vi "Create Event Topics_Latest.vi"() -> (0 "error out":errorcluster, 3 "appended array":string[][](array[string]))   [LabVIEW 2014]
uses:
  <vilib>/National Instruments/NI Amazon Web Services (AWS) Toolkit for LabVIEW/S3/vi source/Typedefs/AMZ_S3_AWS Credentials.ctl
  <vilib>/National Instruments/NI Amazon Web Services (AWS) Toolkit for LabVIEW/SNS/VI Source/Public Typedefs/AWS_SNS CreateTopicParameters.ctl
  <vilib>/National Instruments/NI Amazon Web Services (AWS) Toolkit for LabVIEW/SNS/VI Source/Public Typedefs/AWS_SNS SetTopicAttributes.ctl
  <vilib>/Utility/file.llb/Read From Spreadsheet File (string).vi
  <vilib>/National Instruments/NI Amazon Web Services (AWS) Toolkit for LabVIEW/SNS/VI Source/AWS SNS Class/AWS_SNS.lvclass
  <vilib>/National Instruments/NI Amazon Web Services (AWS) Toolkit for LabVIEW/S3/vi source/LV Interface for Amazon S3.lvlib
  <vilib>/National Instruments/NI Amazon Web Services (AWS) Toolkit for LabVIEW/SNS/VI Source/AWS_SNS.lvlib
panel:
  out "TopicArn":string
  out "resulting string":string
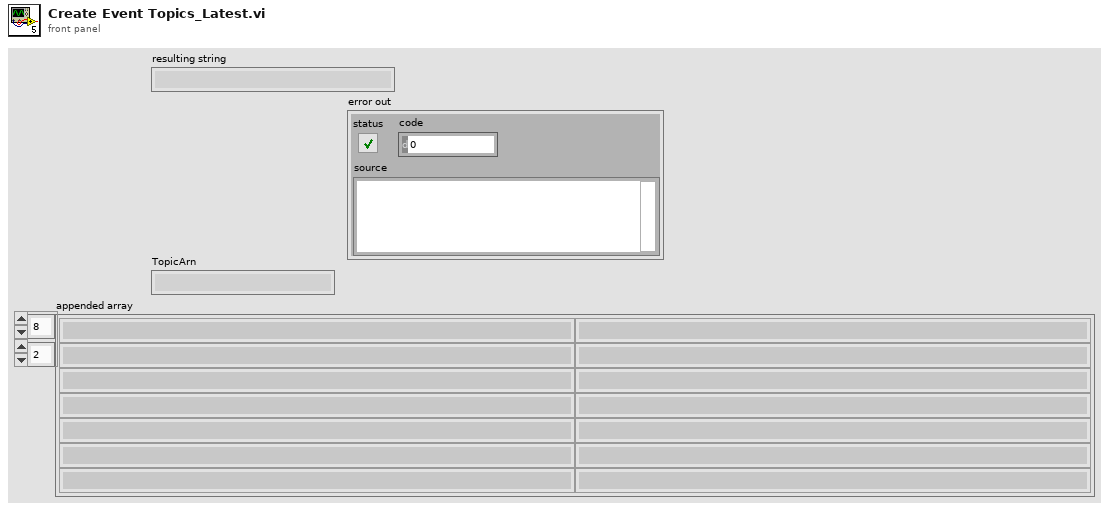
[diagram p1: front panel]
types:
  T1 = typedef "AWS_SNS.lvlib/AWS_SNS CreateTopicParameters.ctl" = string
  T2 = typedef "LV Interface for Amazon S3.lvlib/AMZ_S3_AWS Credentials.ctl" = cluster{"Access Key":string, "Secret Key":string}
  T3 = typedef "AWS_SNS.lvlib/AWS_SNS SetTopicAttributes.ctl" = cluster{"AttributeName":string, "AttributeValue":string, "TopicArn":string}
  T4 = typedef "AWS_SNS.lvlib/CreateTopicResult.ctl" = string
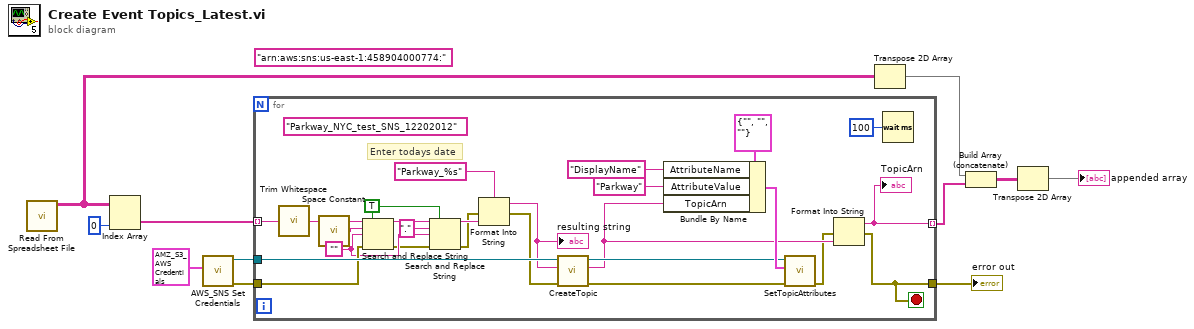
[diagram p0: block diagram]
diagram:
  (unwired) T1 "arn:aws:sns:us-east-1:458904000774:" ("CreateTopic Parameters")
  n1 = call-poly <vilib>:"Read From Spreadsheet File.vi"() -> ("all rows"=w4:string[][])  [unwired: 7 in, 4 out]
  n2 = Index Array(array=w4, index (col)=0 ("disabled index (col)")) -> (element=w6:string[])  [unwired: 1 in]
  n3 = call <vilib>:"AWS_SNS Set Credentials.vi"("AWS Credentials"=T2 {"Access Key"="AKIAIBWID7GQA3ZVLBGQ", "Secret Key"="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"} ("AWS Credentials in")) -> ("error out"=w8:errorcluster, "AWS_SNS.lvlib:AWS_SNS.lvclass"=w9:refnum<class "AWS_SNS.lvclass">)  [unwired: 9 in]
  n4 = for {
    tunnel: w6 -> [w31] mode=indexing
    tunnel: w9 -> [w32]
    tunnel: w8 -> [w26]
    tunnel: [w13] -> w7
    tunnel: [w15] -> w5 mode=indexing
    stop <- w13 stop-if-true
    w23 = ""
    w21 = TRUE ("replace all? (F)")
    (unwired) T1 "Parkway_NYC_test_SNS_12202012" ("CreateTopic Parameters")
    # "Enter todays date"
    n5 = call <vilib>:"Trim Whitespace.vi"("string"=w31) -> ("trimmed string"=w28:string)  [unwired: 1 in]
    n6 = call <vilib>:"Space Constant.vi"() -> ("String"=w27:string)
    n7 = Search and Replace String(replace all?=w21, input string=w28, search string=w27, replace string=w23, error in=w26) -> (result string=w24:string, error out=w18:errorcluster)  [unwired: 3 in, 2 out]
    n8 = Search and Replace String(replace all?=w21, input string=w24, search string=".", replace string=w23, error in=w18) -> (result string=w20:string, error out=w17:errorcluster)  [unwired: 3 in, 2 out]
    n9 = Format Into String(format string="Parkway_%s", error in=w17, w20) -> (resulting string=w29:string, error out=w25:errorcluster)  [unwired: 1 in]
    "resulting string" <- w29
    n10 = call-dynamic "CreateTopic.vi"("error in (no error)"=w25, "CreateTopic Parameters"=w29, "AWS_SNS in"=w32) -> ("error out"=w34:errorcluster, "TopicArn"=w16:T4, "AWS_SNS out"=w33:refnum<class "AWS_SNS.lvclass">)  [unwired: 6 in]
    n11 = Bundle By Name(cluster=T3 {"AttributeName"="", "AttributeValue"="", "TopicArn"=""} ("SetTopicAttributes Parameters"), "AttributeName"="DisplayName", "AttributeValue"="Parkway" ("trimmed string"), "TopicArn"=w16) -> (w36:T3)
    n12 = call-dynamic "SetTopicAttributes.vi"("error in (no error)"=w34, "SetTopicAttributes Parameters"=w36, "AWS_SNS.lvlib:AWS_SNS.lvclass"=w33) -> ("error out"=w14:errorcluster)  [unwired: 7 in, 1 out]
    n13 = Format Into String(error in=w14, w16) -> (resulting string=w15:string, error out=w13:errorcluster)  [unwired: 2 in]
    "TopicArn" <- w15
    n14 = Wait (ms)(milliseconds to wait=u32 100) -> ()  [unwired: 1 out]
  }
  "error out" <- w7
  n15 = Transpose 2D Array(2D array=w4) -> (transposed array=w3:string[][])
  n16 = Build Array (concatenate)(w3, w5) -> (w2:string[][])
  n17 = Transpose 2D Array(2D array=w2) -> (transposed array=→"appended array":string[][])
